vi "controlRtOutMode.vi"(7 "set":bool, 8 "error in":errorcluster, 9 "RtOutMode":enum16{"Off", "AquadB", "Trigger"}(ring), 10 "axis":i32, 11 "connection ID":i32) -> (0 "error out":errorcluster, 1 "RtOutMode":enum16{"Off", "AquadB", "Trigger"}(ring), 2 "axis_out":i32, 3 "connection ID":i32)   [LabVIEW 2016]
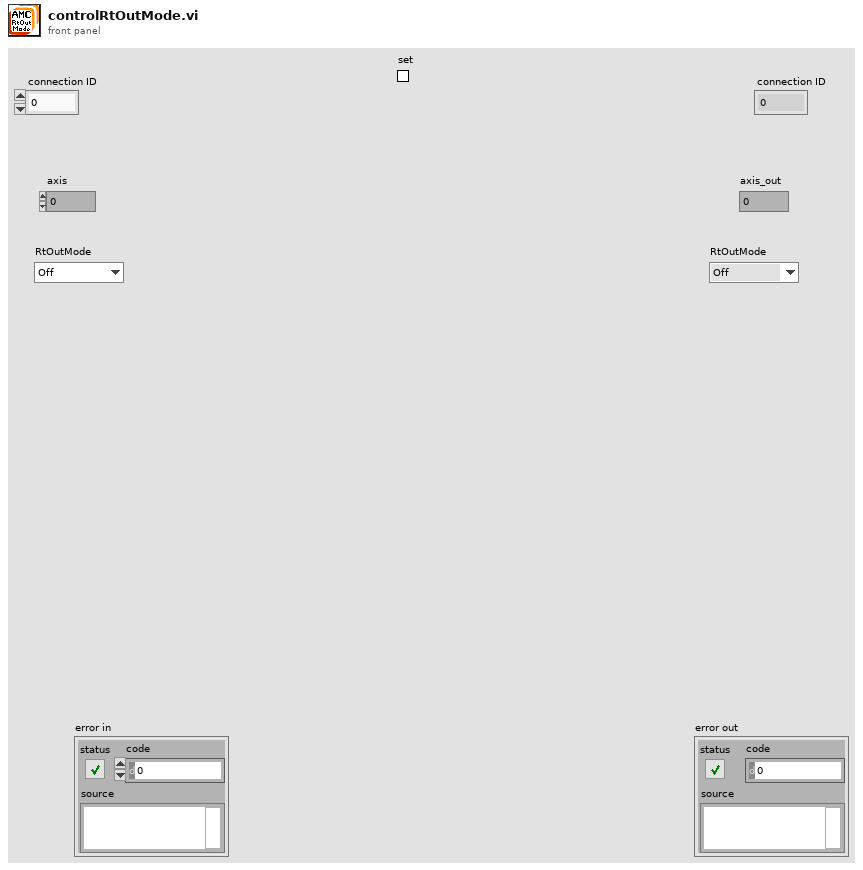
[diagram p1: front panel]
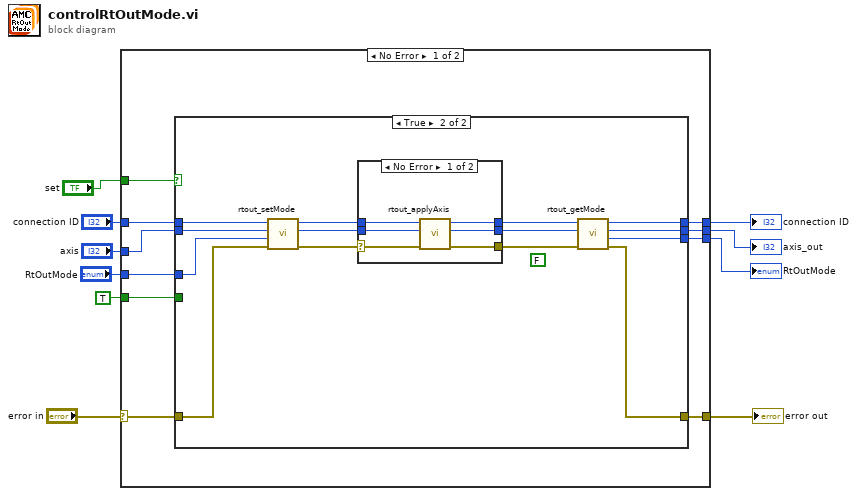
[diagram p0: block diagram]
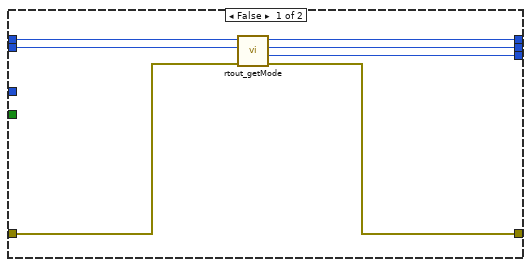
[diagram p2: hidden frame]
diagram:
  n1 = case shown="No Error" "error in" {
    selector: "error in" -> [w13 w54]
    tunnel: [w14 w54] -> w10
    tunnel: [w18 w53] -> w9
    tunnel: "connection ID" -> [w19 w53]
    tunnel: "axis" -> [w16 w52]
    tunnel: TRUE ("tempvalue") -> [w17 _]
    tunnel: [w12 w51] -> w4
    tunnel: "set" -> [w20 _]
    tunnel: [w15 w52] -> w2
    tunnel: "RtOutMode" -> [w11 w51]
    frame No Error {
      n2 = case shown="True" w20 {
        tunnel: w19 -> [w27 w41]
        tunnel: [w26 w33] -> w18
        tunnel: w17 -> [_ _]
        tunnel: w16 -> [w25 w39]
        tunnel: [w24 w29] -> w15
        tunnel: [w23 w32] -> w14
        tunnel: w13 -> [w22 w40]
        tunnel: [w21 w28] -> w12
        tunnel: w11 -> [_ w38]
        frame False {
          n3 = call "rtout_getMode.vi"("error in"=w22, "axis"=w25, "connection ID"=w27) -> ("error out"=w23:errorcluster, "mode"=w21:i32, "axis_out"=w24:i32, "connection ID"=w26:i32)  [unwired: 5 in]
        }
        frame True {
          (unwired) FALSE ("tempvalue")
          n4 = call "rtout_setMode.vi"("error in"=w40, "mode"=w38, "axis"=w39, "connection ID"=w41) -> ("error out"=w35:errorcluster, "axis_out"=w36:i32, "connection ID"=w37:i32)  [unwired: 5 in]
          n5 = case shown="No Error" w35 {
            selector: w35 -> [w43 w48]
            tunnel: w37 -> [w47 w50]
            tunnel: w36 -> [w46 w49]
            tunnel: [w45 w50] -> w34
            tunnel: [w44 w49] -> w31
            tunnel: [w42 w48] -> w30
            frame No Error {
              n6 = call "rtout_applyAxis.vi"("error in"=w43, "axis"=w46, "connection ID"=w47) -> ("error out"=w42:errorcluster, "axis_out"=w44:i32, "connection ID"=w45:i32)  [unwired: 6 in]
            }
            frame Error {
            }
          }
          n7 = call "rtout_getMode.vi"("error in"=w30, "axis"=w31, "connection ID"=w34) -> ("error out"=w32:errorcluster, "mode"=w28:i32, "axis_out"=w29:i32, "connection ID"=w33:i32)  [unwired: 5 in]
        }
      }
    }
    frame Error {
    }
  }
  "error out" <- w10
  "connection ID" <- w9
  "axis_out" <- w2
  "RtOutMode" <- w4
